vi "meth.Destructor.vi"(0 "GLue in":refnum<class "class.GLue.lvclass">, 11 "error in":errorcluster, 13 "ms timeout (-1)":i32=-1) -> (15 "error out":errorcluster)   [LabVIEW 2014, in "GLue.lvlib" / "class.GLue.lvclass"]
uses:
  class.GLue.lvclass
  class.GLue.lvclass/class.GLue.ctl
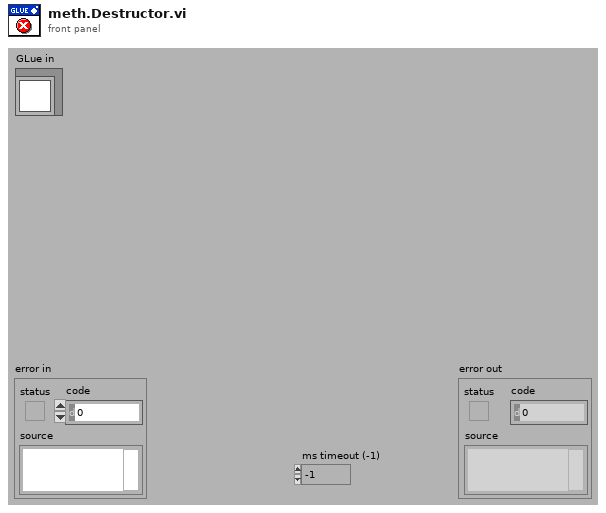
[diagram p1: front panel]
types:
  T1 = typedef "Semaphore RefNum" = refnum<k1>
  T2 = cluster{"StreamReader":refnum<vi>, "UserData":variant}
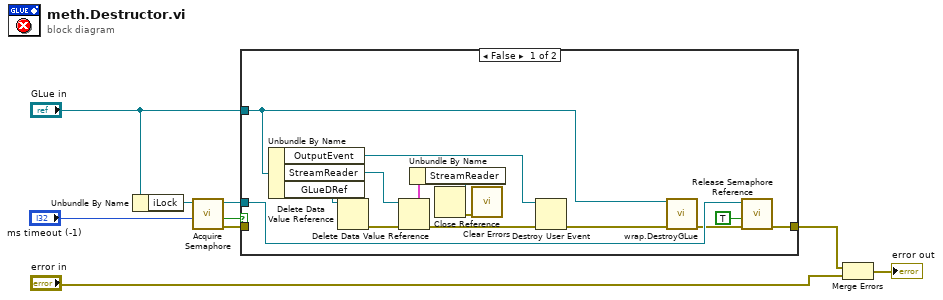
[diagram p0: block diagram]
diagram:
  n1 = Unbundle By Name("GLue in") -> ("iLock"=w9:T1)
  n2 = call <vilib>:"Acquire Semaphore.vi"("ms timeout (-1)"="ms timeout (-1)", "semaphore"=w9) -> ("error out"=w6:errorcluster, "timed out"=w7:bool, "semaphore out"=w5:T1)  [unwired: 3 in]
  n3 = case shown="False" w7 {
    tunnel: w6 -> [_ w24]
    tunnel: w5 -> [w22 _]
    tunnel: "GLue in" -> [w11 _]
    tunnel: [w21 w24] -> w1
    frame False {
      n4 = Unbundle By Name(w11) -> ("OutputEvent"=w16:refnum<user-event>, "StreamReader"=w17:refnum<data-value>, "GLueDRef"=w20:refnum<data-value>)
      n5 = Delete Data Value Reference(data value reference=w20) -> (error out=w18:errorcluster)  [unwired: 1 in, 1 out]
      n6 = Delete Data Value Reference(data value reference=w17, error in=w18) -> (data value=w14:T2, error out=w15:errorcluster)
      n7 = Unbundle By Name(w14) -> ("StreamReader"=w13:refnum<vi>)
      n8 = Close Reference(reference=w13) -> (error out=w12:errorcluster)  [unwired: 1 in]
      n9 = call <vilib>:"Clear Errors.vi"("error in (no error)"=w12) -> ()  [unwired: 5 in, 2 out]
      n10 = Destroy User Event(user event=w16, error in=w15) -> (error out=w10:errorcluster)
      n11 = call "wrap.DestroyGLue.vi"("class.GLue in"=w11, "error in (no error)"=w10) -> ("error out"=w19:errorcluster)  [unwired: 12 in, 1 out]
      n12 = call <vilib>:"Release Semaphore Reference.vi"("error in (no error)"=w19, "force destroy? (F)"=TRUE, "semaphore"=w22) -> ("error out"=w21:errorcluster)  [unwired: 7 in, 1 out]
    }
    frame True {
    }
  }
  n13 = Merge Errors(w1, "error in") -> (→"error out":errorcluster)
